vi "5.11-TCP Send Client.vi"() -> ()   [LabVIEW 2010]
doc: "Displays data sent via TCP from Data Server.vi. Once a TCP connection is open, the VI reads 4 bytes to determine the amount of data being sent. It then reads and charts that many bytes. If an error occurs or the stop button is pressed, it sends a \"Q\" to the Data Sender to notify it to quit.\n\n<B>Note:</B> Requires the Data Server.vi located in the same library as this VI."
uses:
  4-High Neurons/6.1-Forbrain Act Neurons.ctl
  4-High Neurons/4.1.2-Act Neuron TD.ctl
  4-High Neurons/4.1-Act Control Typedef.ctl
  6-OCU Neurons/6.1-UDP Saitek.ctl
  5.0-Global.vi
panel:
  in  "Address":string="10.10.10.2"
  in  "Port":u16=53483 min=1025 step=1
  # "Instructions:\n1. Open the Data Server.vi located in the same library.\n2. Follow the instructions on it's front panel.\n\nNote: This VI is built to work with the Data Server.vi."
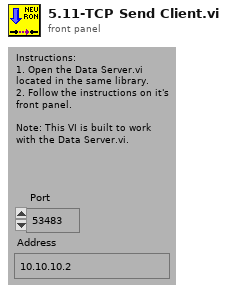
[diagram p1: front panel]
types:
  T1 = typedef "6.1-Forbrain Act Neurons.ctl" = cluster{"Forebrain Act Neurons":T2, "4.1 Act Control":T3}
  T2 = typedef "4.1.2-Act Neuron TD.ctl" = cluster{"Speed By Path":sgl[]}
  T3 = typedef "4.1-Act Control Typedef.ctl" = cluster{"E-Stop":bool, "Restart":bool, "Extended Joystick":bool, "Begin":bool, "Time":i32, "Shutdown":bool, "Saitek Controler":T4, "Joystick Valid":bool}
  T4 = typedef "6.1-UDP Saitek.ctl" = cluster{"Stop":bool, "Setpoint":bool, "Run":bool, "Restart":bool, "Shutdown":bool, "Joystick\nMode 1":bool, "Joystick\nMode 2":bool, "Joystick \nMode 3":bool, "Joystick Mode 4":bool, "10":bool, "11":bool, "Pitch":sgl, "Roll":sgl, "Yaw":sgl, "Left":sgl, "Right":sgl}
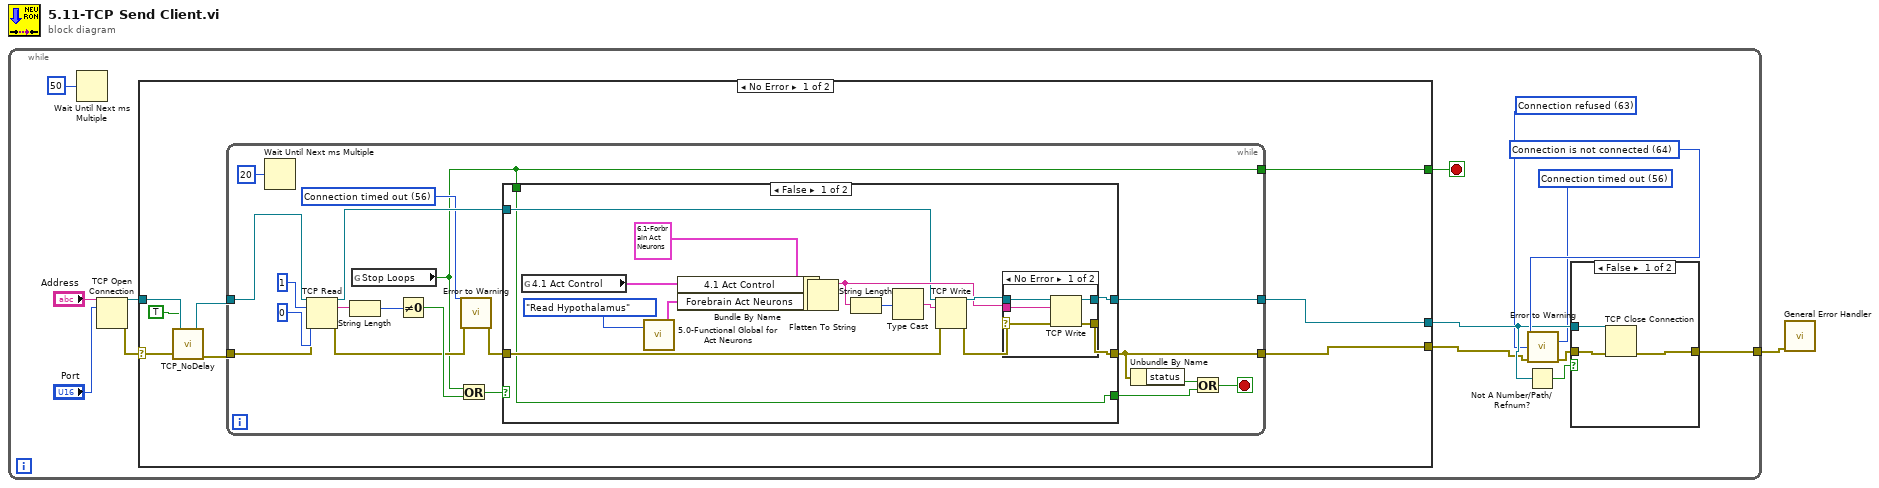
[diagram p0: block diagram]
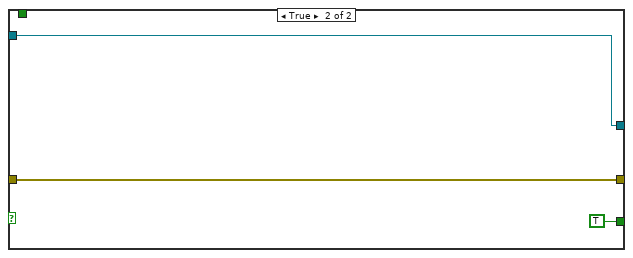
[diagram p4: hidden frame]
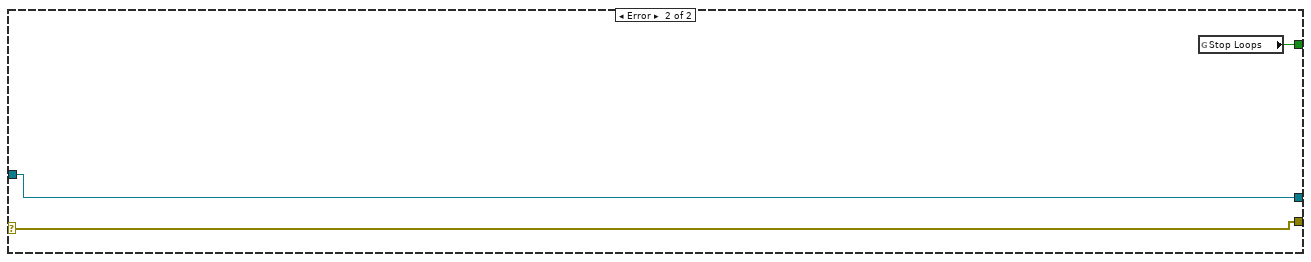
[diagram p5: hidden frame]
diagram:
  n1 = while {
    tunnel: [w4] -> w1
    stop <- w10 stop-if-true
    w2 = 56 items=["No Error", "Argument Error", "Memory Full", "Out of Zone", "End of File", "File Already Open", "Generic File IO Error", "File Not Found", "File Permission Error", "Disk Full", "Duplicate Path", "Too Many Files Open", "Not Enabled", "Resource File Not Found", "Cannot Add Resource", "Resource Not Found", "Image Not Found", "Image Memory Error", "Pen Does Not Exist", "Config Bad Type", "Config Token Not Found", "Config Parse Error", "Config Memory Error", "Bad External Code Format", "Bad External Code Offset", "External Code Not Present", "Null Window", "Destroy Window Mixup", "Null Menu", "Print Aborted", "Bad Print Record", "Print Driver Error", "Windows Error During Print", "Memory Error During Print", "Print Dialog Error", "Generic Print Error", "Invalid Device Refnum", "Device Not Found", "Device Parameter Error", "Device Unit Error", "Can't Open Device", "Device Call Aborted", "Generic Error", "Cancelled By User", "Object ID Too Low", "Object ID Too High", "Object Not In Heap", "Unknown Heap", "Bad DefProc ID", "DefProc Not In Table", "Message Out Of Range", "Null Method", "Unknown Message", "Manager Call Not Supported", "Bad address", "Connection In progress", "Connection timed out", "Connection is already in progress", "Network attribute not supported", "Network error", "Address in use", "System out of memory", "Connection aborted", "Connection refused", "Connection is not connected", "Connection is already connected", "Connection closed", "Initialize error (interapplication manager)", "Bad occurrence", "Wait on unbound occurrence handler", "Occurrence queue overflow", "Bad path", "Semaphore not signaled", "Unrecognized type (interapplication manager)"] ("2nd Error to Convert")
    w3 = 63 items=["No Error", "Argument Error", "Memory Full", "Out of Zone", "End of File", "File Already Open", "Generic File IO Error", "File Not Found", "File Permission Error", "Disk Full", "Duplicate Path", "Too Many Files Open", "Not Enabled", "Resource File Not Found", "Cannot Add Resource", "Resource Not Found", "Image Not Found", "Image Memory Error", "Pen Does Not Exist", "Config Bad Type", "Config Token Not Found", "Config Parse Error", "Config Memory Error", "Bad External Code Format", "Bad External Code Offset", "External Code Not Present", "Null Window", "Destroy Window Mixup", "Null Menu", "Print Aborted", "Bad Print Record", "Print Driver Error", "Windows Error During Print", "Memory Error During Print", "Print Dialog Error", "Generic Print Error", "Invalid Device Refnum", "Device Not Found", "Device Parameter Error", "Device Unit Error", "Can't Open Device", "Device Call Aborted", "Generic Error", "Cancelled By User", "Object ID Too Low", "Object ID Too High", "Object Not In Heap", "Unknown Heap", "Bad DefProc ID", "DefProc Not In Table", "Message Out Of Range", "Null Method", "Unknown Message", "Manager Call Not Supported", "Bad address", "Connection In progress", "Connection timed out", "Connection is already in progress", "Network attribute not supported", "Network error", "Address in use", "System out of memory", "Connection aborted", "Connection refused", "Connection is not connected", "Connection is already connected", "Connection closed", "Initialize error (interapplication manager)", "Bad occurrence", "Wait on unbound occurrence handler", "Occurrence queue overflow", "Bad path", "Semaphore not signaled", "Unrecognized type (interapplication manager)"] ("3rd Error to Convert")
    w9 = 64 items=["No Error", "Argument Error", "Memory Full", "Out of Zone", "End of File", "File Already Open", "Generic File IO Error", "File Not Found", "File Permission Error", "Disk Full", "Duplicate Path", "Too Many Files Open", "Not Enabled", "Resource File Not Found", "Cannot Add Resource", "Resource Not Found", "Image Not Found", "Image Memory Error", "Pen Does Not Exist", "Config Bad Type", "Config Token Not Found", "Config Parse Error", "Config Memory Error", "Bad External Code Format", "Bad External Code Offset", "External Code Not Present", "Null Window", "Destroy Window Mixup", "Null Menu", "Print Aborted", "Bad Print Record", "Print Driver Error", "Windows Error During Print", "Memory Error During Print", "Print Dialog Error", "Generic Print Error", "Invalid Device Refnum", "Device Not Found", "Device Parameter Error", "Device Unit Error", "Can't Open Device", "Device Call Aborted", "Generic Error", "Cancelled By User", "Object ID Too Low", "Object ID Too High", "Object Not In Heap", "Unknown Heap", "Bad DefProc ID", "DefProc Not In Table", "Message Out Of Range", "Null Method", "Unknown Message", "Manager Call Not Supported", "Bad address", "Connection In progress", "Connection timed out", "Connection is already in progress", "Network attribute not supported", "Network error", "Address in use", "System out of memory", "Connection aborted", "Connection refused", "Connection is not connected", "Connection is already connected", "Connection closed", "Initialize error (interapplication manager)", "Bad occurrence", "Wait on unbound occurrence handler", "Occurrence queue overflow", "Bad path", "Semaphore not signaled", "Unrecognized type (interapplication manager)"] ("1st Error to Convert")
    n2 = Wait Until Next ms Multiple(millisecond multiple=u32 50) -> ()  [unwired: 1 out]
    n3 = TCP Open Connection(address="Address", remote port or service name="Port") -> (connection ID=w13:refnum<k5>, error out=w12:errorcluster)  [unwired: 1 in, 2 out]
    n4 = case shown="No Error" w12 {
      selector: w12 -> [w23 w72]
      tunnel: w13 -> [w26 w73]
      tunnel: [w27 w74] -> w10
      tunnel: [w21 w73] -> w6
      tunnel: [w20 w72] -> w5
      frame No Error {
        n5 = call "TCP_NoDelay.vi"("error in (no error)"=w23, "TCP_NODELAY (true)"=TRUE, "connID"=w26) -> ("error out"=w24:errorcluster, "connID 2"=w25:refnum<k5>)  [unwired: 3 in]
        n6 = while {
          tunnel: [w29] -> w27
          tunnel: [w38] -> w20
          tunnel: w25 -> [w31]
          tunnel: [w33] -> w21
          tunnel: w24 -> [w32]
          stop <- w46 stop-if-true
          w36 = 56 items=["No Error", "Argument Error", "Memory Full", "Out of Zone", "End of File", "File Already Open", "Generic File IO Error", "File Not Found", "File Permission Error", "Disk Full", "Duplicate Path", "Too Many Files Open", "Not Enabled", "Resource File Not Found", "Cannot Add Resource", "Resource Not Found", "Image Not Found", "Image Memory Error", "Pen Does Not Exist", "Config Bad Type", "Config Token Not Found", "Config Parse Error", "Config Memory Error", "Bad External Code Format", "Bad External Code Offset", "External Code Not Present", "Null Window", "Destroy Window Mixup", "Null Menu", "Print Aborted", "Bad Print Record", "Print Driver Error", "Windows Error During Print", "Memory Error During Print", "Print Dialog Error", "Generic Print Error", "Invalid Device Refnum", "Device Not Found", "Device Parameter Error", "Device Unit Error", "Can't Open Device", "Device Call Aborted", "Generic Error", "Cancelled By User", "Object ID Too Low", "Object ID Too High", "Object Not In Heap", "Unknown Heap", "Bad DefProc ID", "DefProc Not In Table", "Message Out Of Range", "Null Method", "Unknown Message", "Manager Call Not Supported", "Bad address", "Connection In progress", "Connection timed out", "Connection is already in progress", "Network attribute not supported", "Network error", "Address in use", "System out of memory", "Connection aborted", "Connection refused", "Connection is not connected", "Connection is already connected", "Connection closed", "Initialize error (interapplication manager)", "Bad occurrence", "Wait on unbound occurrence handler", "Occurrence queue overflow", "Bad path", "Semaphore not signaled", "Unrecognized type (interapplication manager)"] ("1st Error to Convert")
          n7 = Wait Until Next ms Multiple(millisecond multiple=u32 20) -> ()  [unwired: 1 out]
          n8 = TCP Read(connection ID=w31, bytes to read=1, error in (no error)=w32, 9:0) -> (connection ID out=w42:refnum<k5>, data out=w43:string, error out=w35:errorcluster)  [unwired: 1 in]
          n9 = String Length(string=w43) -> (length=w41:i32)
          n10 = global read "5.0-Global.vi" "Stop Loops"() -> (w29:bool)
          n11 = Not Equal To 0?(x=w41) -> (x != 0?=w40:bool)
          n12 = Or(x=w29, y=w40) -> (x .or. y?=w39:bool)
          n13 = call <vilib>:"Error to Warning.vi"("1st Error to Convert"=w36, "error in"=w35) -> ("warning out"=w34:errorcluster)  [unwired: 13 in]
          n14 = case shown="False" w39 {
            tunnel: w34 -> [w58 w69]
            tunnel: w42 -> [w54 w70]
            tunnel: [w57 w70] -> w33
            tunnel: [w56 w69] -> w38
            tunnel: [w47 TRUE] -> w28
            tunnel: w29 -> [w47 _]
            frame False {
              n15 = global read "5.0-Global.vi" "4.1 Act Control"() -> (w51:T3)
              n16 = call "5.0-Functional Global for Act Neurons.vi"("Mode"=enum16{"Set Hypothalamus", "Read Hypothalamus"}."Read Hypothalamus") -> ("Output Act Neurons"=w49:T2)  [unwired: 1 in]
              n17 = Bundle By Name(cluster=T1 {"Forebrain Act Neurons"={"Speed By Path"=[]}, "4.1 Act Control"={"E-Stop"=FALSE, "Restart"=FALSE, "Extended Joystick"=FALSE, "Begin"=FALSE, "Time"=0, "Shutdown"=FALSE, "Saitek Controler"={"Stop"=FALSE, "Setpoint"=FALSE, "Run"=FALSE, "Restart"=FALSE, "Shutdown"=FALSE, "Joystick\nMode 1"=FALSE, "Joystick\nMode 2"=FALSE, "Joystick \nMode 3"=FALSE, "Joystick Mode 4"=FALSE, "10"=FALSE, "11"=FALSE, "Pitch"=0.0, "Roll"=0.0, "Yaw"=0.0, "Left"=0.0, "Right"=0.0}, "Joystick Valid"=FALSE}} ("6.1-Act Neuron"), "4.1 Act Control"=w51, "Forebrain Act Neurons"=w49) -> (w52:T1)
              n18 = Flatten To String(anything=w52) -> (data string=w55:string)  [unwired: 3 in, 2 out]
              n19 = String Length(string=w55) -> (length=w60:i32)
              n20 = Type Cast(x=w60) -> (*(type *) &x=w61:string)  [unwired: 1 in]
              n21 = TCP Write(connection ID=w54, data in=w61, error in (no error)=w58) -> (connection ID out=w59:refnum<k5>, error out=w53:errorcluster)  [unwired: 1 in, 1 out]
              n22 = case shown="No Error" w53 {
                selector: w53 -> [w64 w67]
                tunnel: w59 -> [w66 w68]
                tunnel: [w62 w68] -> w57
                tunnel: [w63 w67] -> w56
                tunnel: w55 -> [w65 _]
                frame No Error {
                  n23 = TCP Write(connection ID=w66, data in=w65, error in (no error)=w64) -> (connection ID out=w62:refnum<k5>, error out=w63:errorcluster)  [unwired: 1 in, 1 out]
                }
                frame Error {
                }
              }
            }
            frame True {
            }
          }
          n24 = Unbundle By Name(w38) -> ("status"=w37:bool)
          n25 = Or(x=w37, y=w28) -> (x .or. y?=w46:bool)
        }
      }
      frame Error {
        n26 = global read "5.0-Global.vi" "Stop Loops"() -> (w74:bool)
      }
    }
    n27 = Not A Number/Path/Refnum?(number/path/refnum=w6) -> (NaN/Path/Refnum?=w8:bool)
    n28 = call <vilib>:"Error to Warning.vi"("1st Error to Convert"=w9, "2nd Error to Convert"=w2, "3rd Error to Convert"=w3, "error in"=w5) -> ("warning out"=w7:errorcluster)  [unwired: 11 in]
    n29 = case shown="False" w8 {
      tunnel: w6 -> [w18 _]
      tunnel: w7 -> [w17 w19]
      tunnel: [w16 w19] -> w4
      frame False {
        n30 = TCP Close Connection(connection ID=w18, error in (no error)=w17) -> (error out=w16:errorcluster)  [unwired: 2 out]
      }
      frame True {
      }
    }
  }
  n31 = call <vilib>:"General Error Handler.vi"("error in (no error)"=w1) -> ()  [unwired: 2 in, 13 out]
